vi "Simple AAP.vi"() -> ()   [LabVIEW 2014]
panel:
  out "Waveform Graph":dynamicdata(graph)
  out "Average Value":dbl
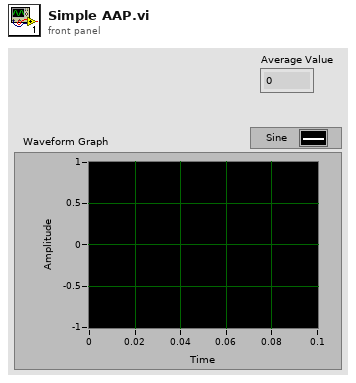
[diagram p1: front panel]
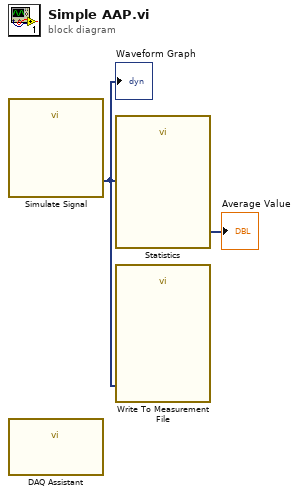
[diagram p0: block diagram]
diagram:
  n1 = call "Simulate Signal"() -> ("Sine"=w1:dynamicdata)  [unwired: 14 in, 1 out]
  "Waveform Graph" <- w1
  n2 = call "DAQ Assistant"() -> ()  [unwired: 12 in]
  n3 = call "Statistics"("Signals"=w1) -> ("Arithmetic Mean"=→"Average Value":dynamicdata)  [unwired: 25 in, 1 out]
  n4 = call "Write To Measurement File"("Signals"=w1) -> ()  [unwired: 16 in, 3 out]
